vi "CAN GIP sample.vi"(8 "error in":errorcluster) -> (0 "error out":errorcluster, 3 "output":dbl[](array[numeric])=[3.0, 3.0, 3.0, 3.0, 3.0, 3.0, 3.0, 3.0, 3.0, 3.0, 3.0, 3.0, 3.0, 3.0, 3.0, 3.0, 3.0, 3.0, 3.0, 3.0, 3.0, 3.0, 3.0, 3.0, 3.0, 3.0, 3.0, 3.0, 3.0, 3.0, 3.0, 3.0, 3.0, 3.0, 3.0, 3.0, 3.0, 3.0, 3.0, 3.0])   [LabVIEW 2021]
uses:
  CAN GIP.lvlib
  Private Controls/CAN States.ctl
  Private Controls/Setting.ctl
panel:
  in  "Input Write":dbl=1.0
  in  "Command":string="GIP_TestMode.GIP_TestModeFlag"
  in  "Write":bool
  in  "Stop Button":bool
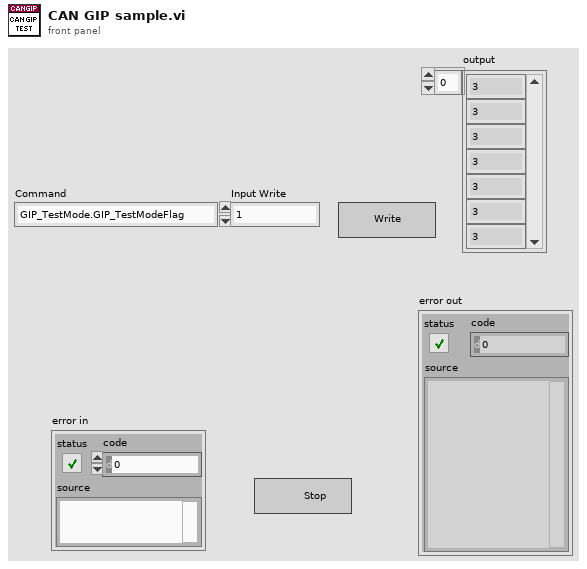
[diagram p1: front panel]
types:
  T1 = typedef "CAN GIP.lvlib/Setting.ctl" = cluster{"Termination":u32, "Baud Rate":u64, "Interface":refnum<k21>, "XNET Database":refnum<k21>, "ECU":refnum<k21>}
  T2 = typedef "CAN GIP.lvlib/CAN States.ctl" = enum16{"Init", "Config", "Read Signals", "Write Signals", "Close"}
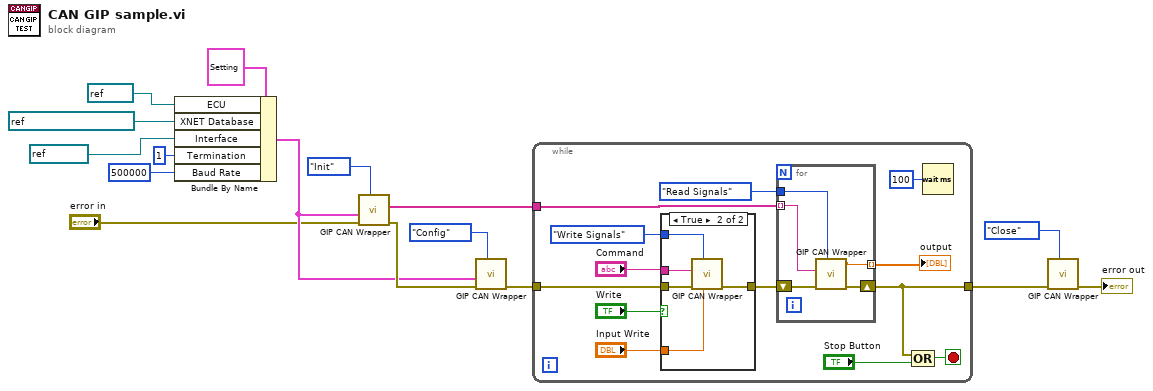
[diagram p0: block diagram]
diagram:
  n1 = Bundle By Name(cluster=T1 {"Termination"=1, "Baud Rate"=125000, "Interface"="CAN1", "XNET Database"="GIP_CAN_Database", "ECU"="GIP\nGIP_CAN_Database"} ("Setting"), "ECU"=refnum<k21> "GIP\ncan_messages_818", "XNET Database"=refnum<k21> "can_messages_818", "Interface"=refnum<k21> "CAN4", "Termination"=u32 1, "Baud Rate"=u64 500000) -> (w10:T1)
  n2 = call "GIP CAN Wrapper.vi"("States"=CAN_States."Init" ("CAN States"), "error in"="error in", "Setting"=w10) -> ("error out"=w15:errorcluster, "Rx SigNames"=w1:string[])  [unwired: 6 in, 1 out]
  n3 = call "GIP CAN Wrapper.vi"("States"=CAN_States."Config" ("CAN States"), "error in"=w15, "Setting"=w10) -> ("error out"=w9:errorcluster)  [unwired: 6 in, 2 out]
  n4 = while {
    tunnel: [w25] -> w8
    tunnel: w9 -> [w21]
    tunnel: w1 -> [w17]
    stop <- w26 stop-if-true
    n5 = case shown="True" "Write" {
      tunnel: [w30 w35] -> w22
      tunnel: CAN_States."Write Signals" ("CAN States") -> [_ w34]
      tunnel: "Command" -> [_ w33]
      tunnel: w21 -> [w30 w32]
      tunnel: "Input Write" -> [_ w31]
      frame False {
      }
      frame True {
        n6 = call "GIP CAN Wrapper.vi"("Signal Write"=w31, "States"=w34, "error in"=w32, "Tx Signal In"=w33) -> ("error out"=w35:errorcluster)  [unwired: 5 in, 2 out]
      }
    }
    n7 = for {
      tunnel: CAN_States."Read Signals" ("CAN States") -> [w40]
      shift-right: [w38] -> w25
      shift-left: w22 -> [w39]
      tunnel: [w37] -> w24 mode=indexing
      tunnel: w17 -> [w36] mode=indexing
      n8 = call "GIP CAN Wrapper.vi"("States"=w40, "error in"=w39, "Tx Signal In"=w36) -> ("error out"=w38:errorcluster, "Signal out"=w37:dbl)  [unwired: 6 in, 1 out]
    }
    "output" <- w24
    n9 = Compound Arithmetic op=OR(w25, "Stop Button") -> (w26:bool)
    n10 = Wait (ms)(milliseconds to wait=u32 100) -> ()  [unwired: 1 out]
  }
  n11 = call "GIP CAN Wrapper.vi"("States"=CAN_States."Close" ("CAN States"), "error in"=w8) -> ("error out"=→"error out":errorcluster)  [unwired: 7 in, 2 out]
